vi "Initialise.vi"(8 "error in (no error)":errorcluster, 10 "Behaviour Tree":refnum<class "bt_Node.lvclass">, 11 "bt_System in":refnum<class "bt_System.lvclass">) -> (0 "error out":errorcluster, 3 "bt_System out":refnum<class "bt_System.lvclass">)   [LabVIEW 2021, in "BT.lvlib" / "bt_System.lvclass"]
uses:
  bt_System.lvclass
  Support/Nodes/abs_Node/bt_Node.lvclass
  bt_System.lvclass/bt_System.ctl
  Properties/Write Behaviour Tree.vi
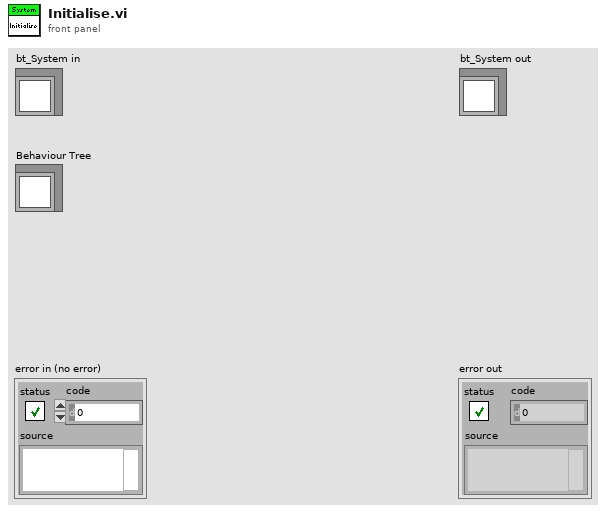
[diagram p1: front panel]
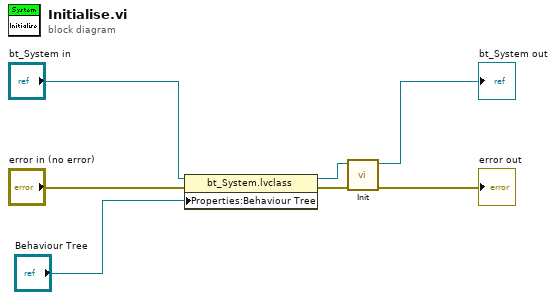
[diagram p0: block diagram]
diagram:
  n1 = property class="bt_System.lvclass"(reference="bt_System in", error in="error in (no error)", "Properties:Behaviour Tree"="Behaviour Tree") -> (reference out=w2:refnum<class "bt_System.lvclass">, error out=w3:errorcluster)
  n2 = call "Init.vi"("error in (no error)"=w3, "bt_System in"=w2) -> ("error out"=→"error out":errorcluster, "bt_System out"=→"bt_System out":refnum<class "bt_System.lvclass">)  [unwired: 8 in]
